vi "InitTable.vi"() -> (0 "Enum out":T1, 3 "HealthCheck out":refnum<class "HealthCheck.lvclass">)   [LabVIEW 2018, in "HealthCheck.lvclass"]
uses:
  HealthCheck.lvclass
  HCState_TypeDef.ctl
  ModifyTableEntry.vi
panel:
  out "error out":errorcluster
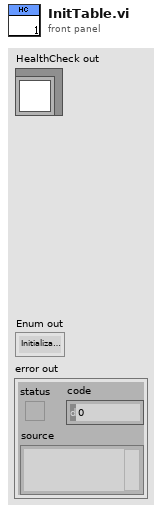
[diagram p1: front panel]
types:
  T1 = typedef "HealthCheck.lvclass/HCState_TypeDef.ctl" = enum16{"Initialization", "Running", "Modify Table"}
  T2 = enum32{"Invalid", "Standard", "Closed", "Hidden", "Minimized", "Maximized"}
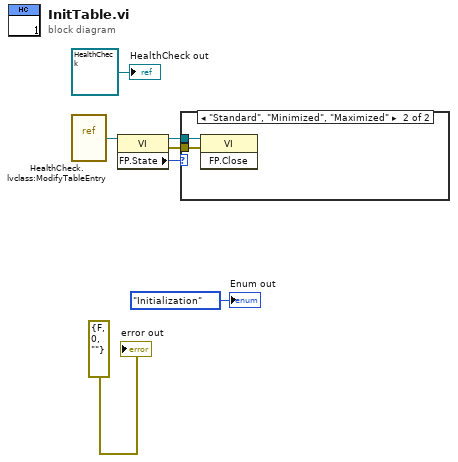
[diagram p0: block diagram]
diagram:
  n1 = vi-ref "HealthCheck.lvclass:ModifyTableEntry.vi"() -> (w5:refnum<vi>)
  n2 = property class="VI"(reference=w5) -> (reference out=w3:refnum<vi>, error out=w2:errorcluster, "FP.State"=w4:T2)  [unwired: 1 in]
  n3 = case shown="\"Standard\", \"Minimized\", \"Maximized\"" w4 {
    tunnel: w3 -> [_ w9]
    tunnel: w2 -> [_ w8]
    frame Default {
    }
    frame "Standard", "Minimized", "Maximized" {
      n4 = invoke class="VI" method="FP.Close"(reference=w9, error in=w8) -> ()  [unwired: 1 in, 3 out]
    }
  }
  "error out" <- errorcluster {"status"=FALSE, "code"=0, "source"=""} ("error out")
  "HealthCheck out" <- refnum<class "HealthCheck.lvclass"> refnum ("HealthCheck out")
  "Enum out" <- HCState_TypeDef."Initialization" ("Enum out")
